vi "sub_transform3x3submatrix.vi"(11 "puzzle (in)":string[][](array[string])=[["", "1", "", "", "", "", "", ""], ["", "", "6", "", "", "", "6", ""], ["", "", "", "", "6", "", "", ""], ["", "", "", "", "", "", "", ""], ["2", "", "", "6", "7", "", "", "9"], ["", "6", "", "", "", "", "", ""], ["", "6", "", "", "4", "", "", ""], ["", "", "", "", "", "", "", ""], ["", "3", "", "", "2", "", "", "3"]]) -> (3 "transformed submatrix":string[][](array[string]))   [LabVIEW 2018]
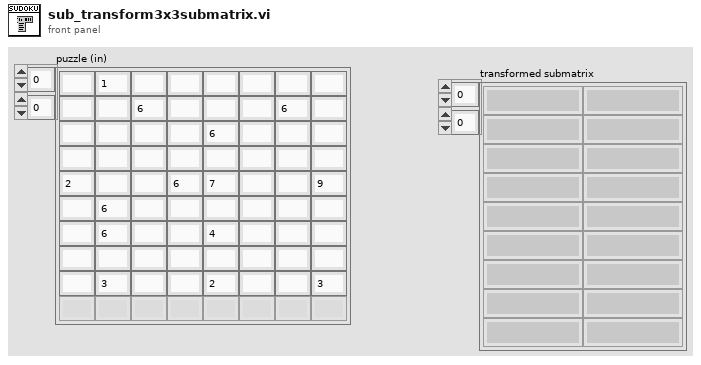
[diagram p1: front panel]
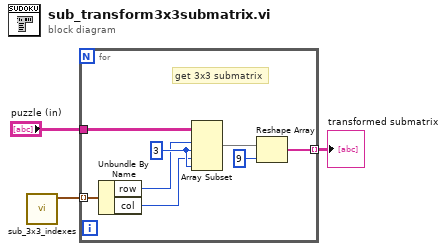
[diagram p0: block diagram]
diagram:
  n1 = call "sub_3x3_indexes.vi"() -> ("3x3 matrix indexes"=w3:cluster{"row":i32, "col":i32}[])  [unwired: 11 in]
  n2 = for {
    tunnel: w3 -> [w6] mode=indexing
    tunnel: "puzzle (in)" -> [w5]
    tunnel: [w4] -> w1 mode=indexing
    w11 = 3 ("length")
    # "get 3x3 submatrix"
    n3 = Unbundle By Name(w6) -> ("row"=w8:i32, "col"=w7:i32)
    n4 = Array Subset(array=w5, index (row)=w8, length (row)=w11, index (col)=w7, length (col)=w11) -> (w10:string[][])
    n5 = Reshape Array(w10, 9 ("dimension size")) -> (w4:string[])
  }
  "transformed submatrix" <- w1
